vi "unflattenPlaneAngleFromXML.vi"   [LabVIEW 2012, in "UnitsAndXML.lvlib"]
doc: "Generates planeAngle in the unit specified in <B>planeAngleUnitInXML</B> from the data in <B>xmlString</B>, where the source unit is <B>planeAngleUnitInXML</B>. The VI uses <B>planeAngleForType</B> to select the appropriate polymorphic method."
uses:
  <userlib>/Common/UnitsAndXML/UnitsAndXML.lvlib
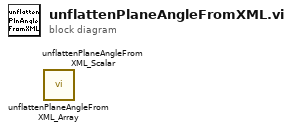
[diagram p0: block diagram]
diagram:
  n1 = call <userlib>:"unflattenPlaneAngleFromXML_Array.vi"() -> ()  [unwired: 10 in, 2 out]
  n2 = call <userlib>:"unflattenPlaneAngleFromXML_Scalar.vi"() -> ()  [unwired: 10 in, 2 out]
